vi "save_base.vi"(0 "Connection In":refnum<k7>, 1 "Url":string(combo), 5 "Error in (no error)":errorcluster) -> (2 "concatenated string":string, 3 "error out":errorcluster, 4 ".not. x?":bool, 6 "Tension":dbl, 7 "Etat":string, 8 "Debit":dbl, 9 "Pression 2":dbl, 10 "Pression":dbl, 11 "Tension2":dbl, 12 "temperature":dbl, 13 "Debit  2":dbl, 14 "Connection Out":refnum<k7>, 15 "Courant":dbl, 16 "temperature 2":dbl, 17 "etat 2":string, 18 "Courant 2":dbl, 19 "Error out":errorcluster)   [LabVIEW 2019]
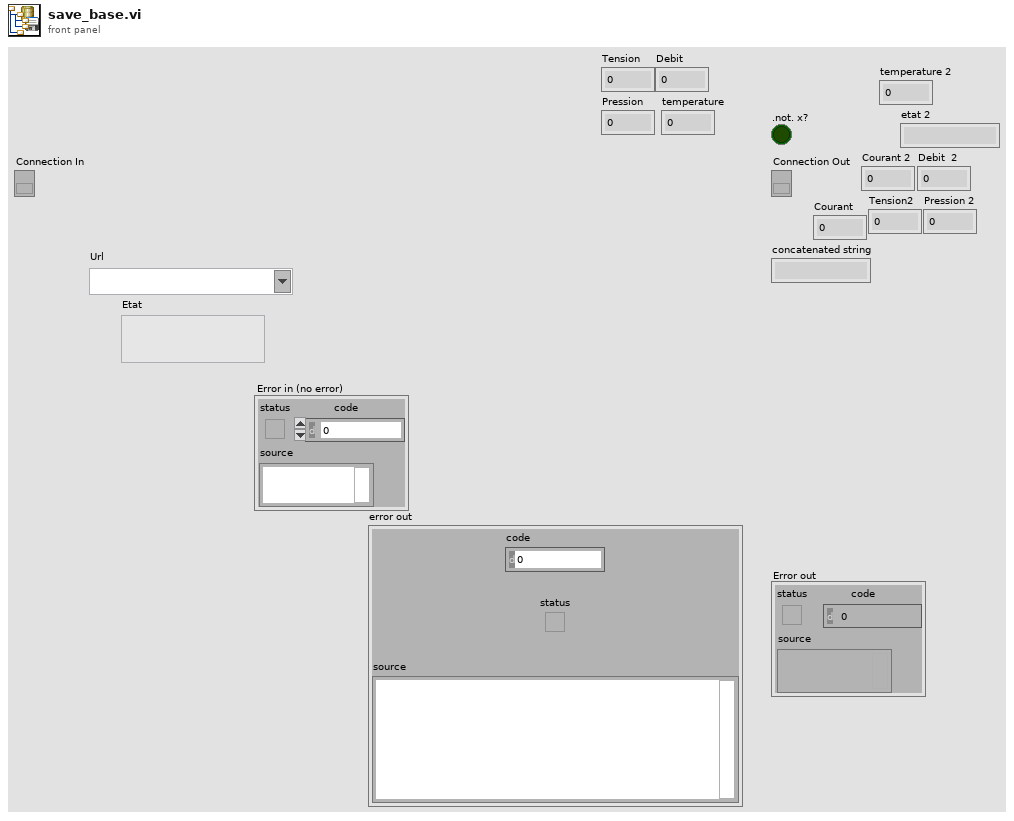
[diagram p1: front panel]
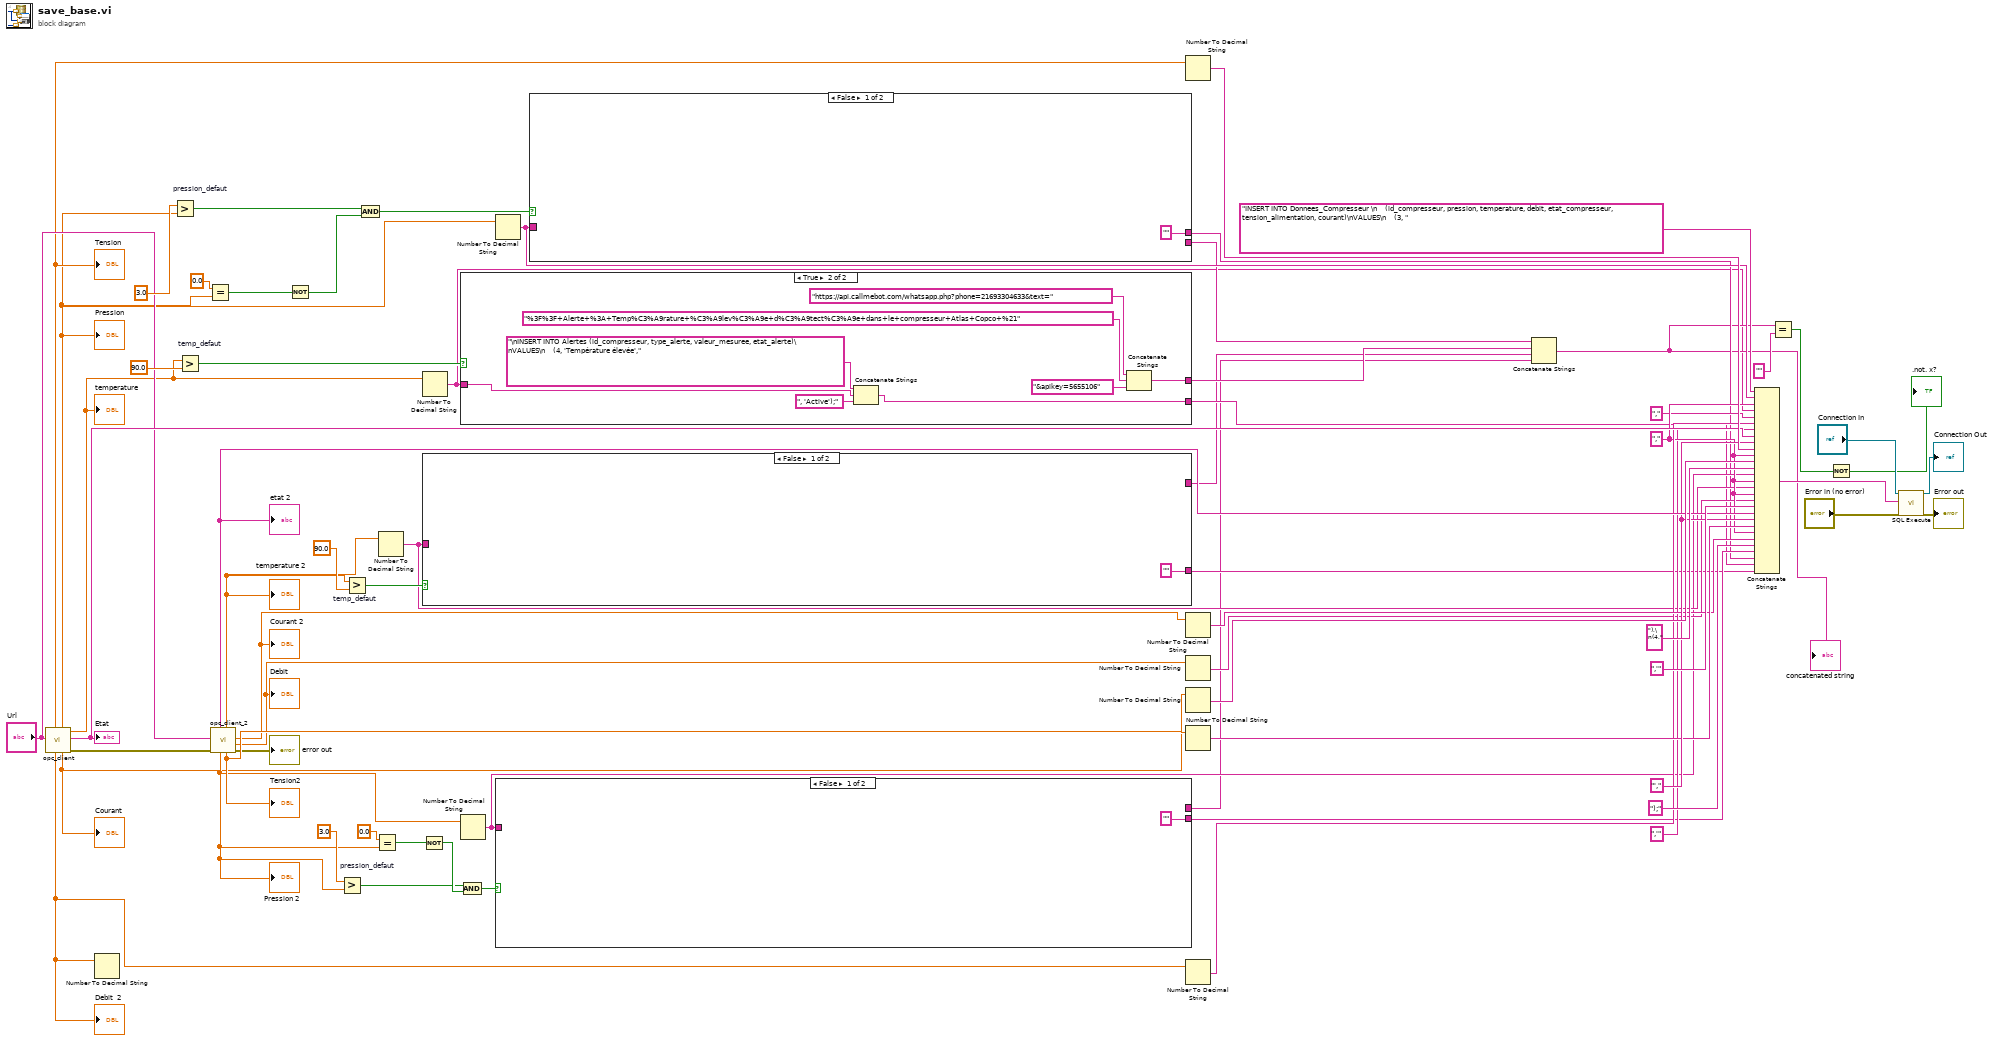
[diagram p0: block diagram]
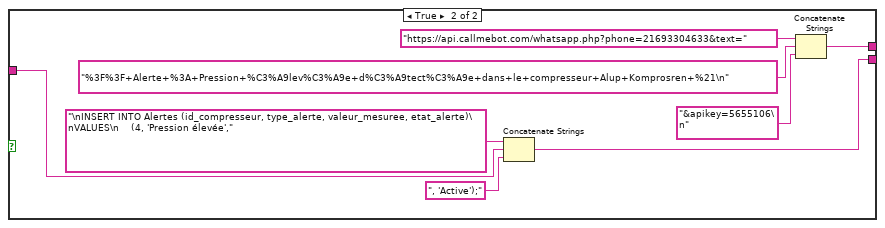
[diagram p2: hidden frame]
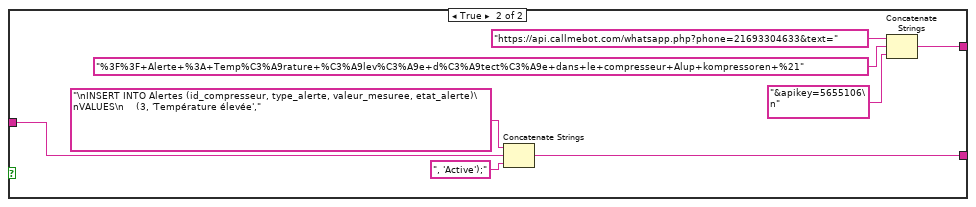
[diagram p3: hidden frame]
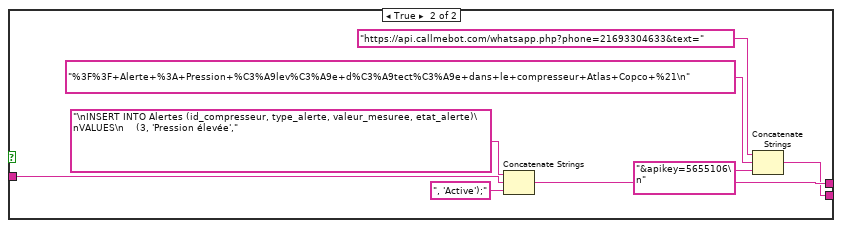
[diagram p4: hidden frame]
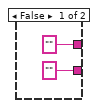
[diagram p5: hidden frame]
diagram:
  w50 = "'," ("string")
  w40 = "," ("string")
  n1 = call "opc_client.vi"("server endpoint URL"="Url") -> ("error out"=w58:errorcluster, "etat"=w53:string, "temperature"=w13:dbl, "Courant"=w11:dbl, "Pression"=w14:dbl, "Debit"=w57:dbl, "Tension"=w15:dbl)  [unwired: 3 in, 1 out]
  "Etat" <- w53
  "Tension" <- w15
  "Pression" <- w14
  "temperature" <- w13
  "Courant" <- w11
  "Debit  2" <- w57
  n2 = Number To Decimal String(number=w57) -> ()  [unwired: 1 in, 1 out]
  n3 = Greater? "pression_defaut"(x=3.0 ("y"), y=w14) -> (0:w63:bool)
  n4 = Greater? "temp_defaut"(x=w13, y=90.0) -> (0:w64:bool)
  n5 = Equal?(x=0.0, y=w14) -> (x = y?=w61:bool)
  n6 = call "opc_client_2.vi"("error in (no error)"=w58, "server endpoint URL"="Url") -> ("error out"=→"error out":errorcluster, "Debit"=w12:dbl, "Courant"=w47:dbl, "Tension"=w49:dbl, "temperature"=w36:dbl, "Pression"=w26:dbl, "etat"=w51:string)  [unwired: 2 in, 1 out]
  "Debit" <- w12
  "temperature 2" <- w36
  "etat 2" <- w51
  "Courant 2" <- w47
  "Tension2" <- w49
  "Pression 2" <- w26
  n7 = Not(x=w61) -> (.not. x?=w60:bool)
  n8 = Greater? "pression_defaut"(x=3.0 ("y"), y=w26) -> (0:w29:bool)
  n9 = Greater? "temp_defaut"(x=w36, y=90.0) -> (0:w35:bool)
  n10 = And(x=w63, y=w60) -> (x .and. y?=w59:bool)
  n11 = Equal?(x=0.0, y=w26) -> (x = y?=w31:bool)
  n12 = Number To Decimal String(number=w36) -> (decimal integer string=w34:string)  [unwired: 1 in]
  n13 = Not(x=w31) -> (.not. x?=w32:bool)
  n14 = Number To Decimal String(number=w13) -> (decimal integer string=w1:string)  [unwired: 1 in]
  n15 = case shown="False" w35 {
    tunnel: ["" w74] -> w21
    tunnel: w34 -> [_ w72]
    tunnel: [_ w69] -> w7
    frame False {
    }
    frame True {
      n16 = Concatenate Strings("\nINSERT INTO Alertes (id_compresseur, type_alerte, valeur_mesuree, etat_alerte)\nVALUES\n    (3, 'Température élevée',", w72, ", 'Active');" ("string")) -> (w74:string)
      n17 = Concatenate Strings("https://api.callmebot.com/whatsapp.php?phone=21693304633&text=" ("string"), "%3F%3F+Alerte+%3A+Temp%C3%A9rature+%C3%A9lev%C3%A9e+d%C3%A9tect%C3%A9e+dans+le+compresseur+Alup+kompressoren+%21" ("string"), "&apikey=5655106\n" ("string")) -> (w69:string)
    }
  }
  n18 = And(x=w29, y=w32) -> (x .and. y?=w27:bool)
  n19 = case shown="True" w64 {
    tunnel: w1 -> [_ w82]
    tunnel: ["" w83] -> w22
    tunnel: ["" w79] -> w8
    frame False {
    }
    frame True {
      n20 = Concatenate Strings("\nINSERT INTO Alertes (id_compresseur, type_alerte, valeur_mesuree, etat_alerte)\nVALUES\n    (4, 'Température élevée',", w82, ", 'Active');" ("string")) -> (w83:string)
      n21 = Concatenate Strings("https://api.callmebot.com/whatsapp.php?phone=21693304633&text=" ("string"), "%3F%3F+Alerte+%3A+Temp%C3%A9rature+%C3%A9lev%C3%A9e+d%C3%A9tect%C3%A9e+dans+le+compresseur+Atlas+Copco+%21" ("string"), "&apikey=5655106" ("string")) -> (w79:string)
    }
  }
  n22 = Number To Decimal String(number=w26) -> (decimal integer string=w25:string)  [unwired: 1 in]
  n23 = Number To Decimal String(number=w14) -> (decimal integer string=w41:string)  [unwired: 1 in]
  n24 = case shown="False" w27 {
    tunnel: w25 -> [_ w91]
    tunnel: ["" w92] -> w24
    tunnel: [_ w88] -> w6
    frame False {
    }
    frame True {
      n25 = Concatenate Strings("\nINSERT INTO Alertes (id_compresseur, type_alerte, valeur_mesuree, etat_alerte)\nVALUES\n    (4, 'Pression élevée',", w91, ", 'Active');" ("string")) -> (w92:string)
      n26 = Concatenate Strings("https://api.callmebot.com/whatsapp.php?phone=21693304633&text=" ("string"), "%3F%3F+Alerte+%3A+Pression+%C3%A9lev%C3%A9e+d%C3%A9tect%C3%A9e+dans+le+compresseur+Alup+Komprosren+%21\n" ("string"), "&apikey=5655106\n" ("string")) -> (w88:string)
    }
  }
  n27 = case shown="False" w59 {
    tunnel: w41 -> [_ w100]
    tunnel: ["" w101] -> w23
    tunnel: [_ w97] -> w9
    frame False {
    }
    frame True {
      n28 = Concatenate Strings("\nINSERT INTO Alertes (id_compresseur, type_alerte, valeur_mesuree, etat_alerte)\nVALUES\n    (3, 'Pression élevée',", w100, ", 'Active');" ("string")) -> (w101:string)
      n29 = Concatenate Strings("https://api.callmebot.com/whatsapp.php?phone=21693304633&text=" ("string"), "%3F%3F+Alerte+%3A+Pression+%C3%A9lev%C3%A9e+d%C3%A9tect%C3%A9e+dans+le+compresseur+Atlas+Copco+%21\n" ("string"), "&apikey=5655106\n" ("string")) -> (w97:string)
    }
  }
  n30 = Number To Decimal String(number=w15) -> (decimal integer string=w56:string)  [unwired: 1 in]
  n31 = Number To Decimal String(number=w47) -> (decimal integer string=w46:string)  [unwired: 1 in]
  n32 = Number To Decimal String(number=w12) -> (decimal integer string=w33:string)  [unwired: 1 in]
  n33 = Number To Decimal String(number=w11) -> (decimal integer string=w55:string)  [unwired: 1 in]
  n34 = Number To Decimal String(number=w49) -> (decimal integer string=w48:string)  [unwired: 1 in]
  n35 = Number To Decimal String(number=w57) -> (decimal integer string=w43:string)  [unwired: 1 in]
  n36 = Concatenate Strings(w9, w8, w7, w6) -> (w4:string)
  "concatenated string" <- w4
  n37 = Concatenate Strings("INSERT INTO Donnees_Compresseur \n    (id_compresseur, pression, temperature, debit, etat_compresseur, tension_alimentation, courant)\nVALUES\n    (3, ", w41, w40, w1, "," ("string"), w43, ",'" ("string"), w53, w50, w56, w40, w55, "),\n(4," ("string"), w25, w40, w34, w40, w33, ",'" ("string"), w51, w50, w48, w40, w46, ");" ("string"), w24, w23, w22, w21) -> (w20:string)
  n38 = Equal?(x=w4, y="") -> (x = y?=w3:bool)
  n39 = Not(x=w3) -> (.not. x?=→".not. x?":bool)
  n40 = call <vilib>:"SQL Execute.vi"("Connection In"="Connection In", "SQL Query"=w20, "Error in (no error)"="Error in (no error)") -> ("Connection Out"=→"Connection Out":refnum<k7>, "Error out"=→"Error out":errorcluster)  [unwired: 15 in]
